vi "label_type_definition.vi"(8 "error_in":errorcluster, 10 "match_scan_code":string, 11 "scan_code":string) -> (0 "error_out":errorcluster, 2 "tooling_name":string, 3 "action":T1)   [LabVIEW 2020]
uses:
  select_action_after_parse.ctl
  control_part_number.ctl
  test_button/FGV_OBJ_test_button.ctl
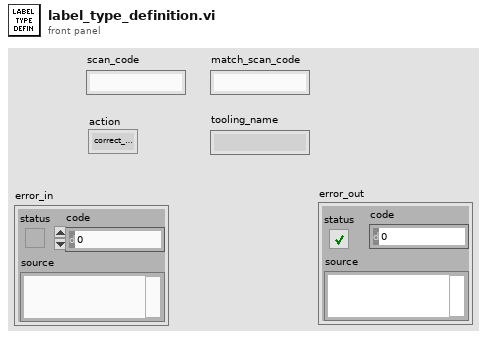
[diagram p1: front panel]
types:
  T1 = typedef "select_action_after_parse.ctl" = enum16{"correct_scan_tooling", "incorrect_scan_tooling", "correct_scan_part", "tooling_and_part_mismatch", "not_scan_tooling"}
  T2 = typedef "control_part_number.ctl" = enum16{"set_parts_number", "get_part_by_name", "set_actual_tool", "get_actual_tool"}
  T3 = typedef "FGV_OBJ_test_button.ctl" = enum16{"initialize", "set_new_login", "set_message", "enable", "disable", "disable_gray", "translate", "set_scan_tooling", "get_scan_tooling"}
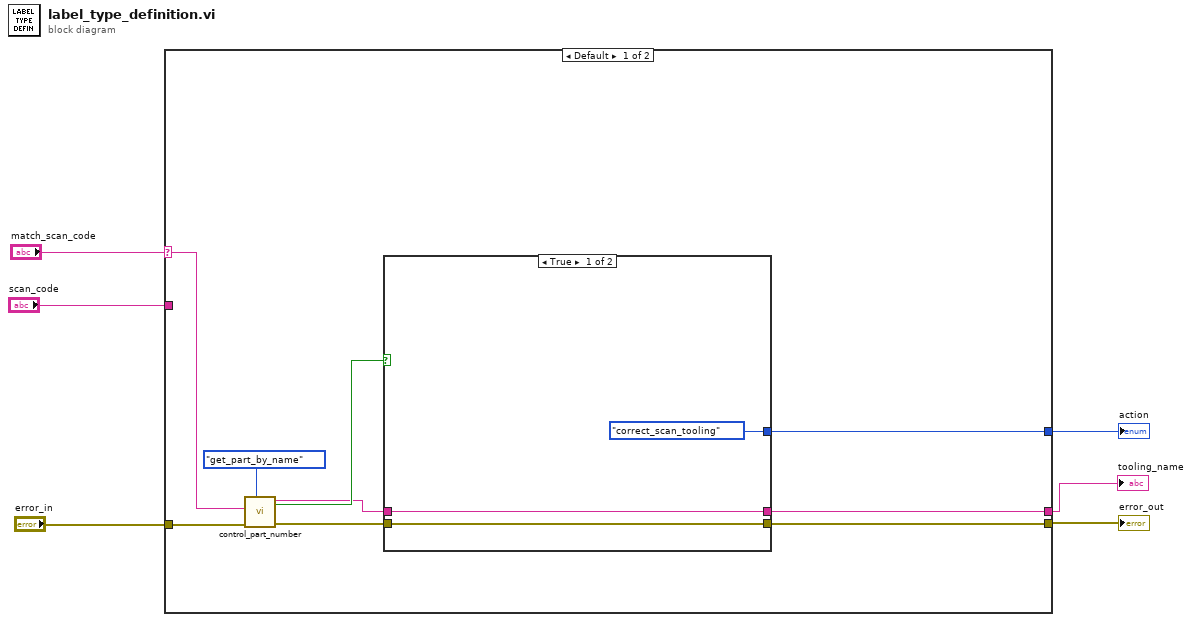
[diagram p0: block diagram]
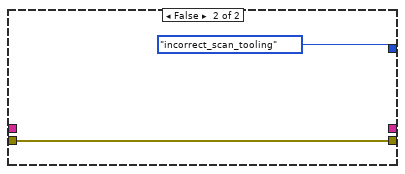
[diagram p2: hidden frame]
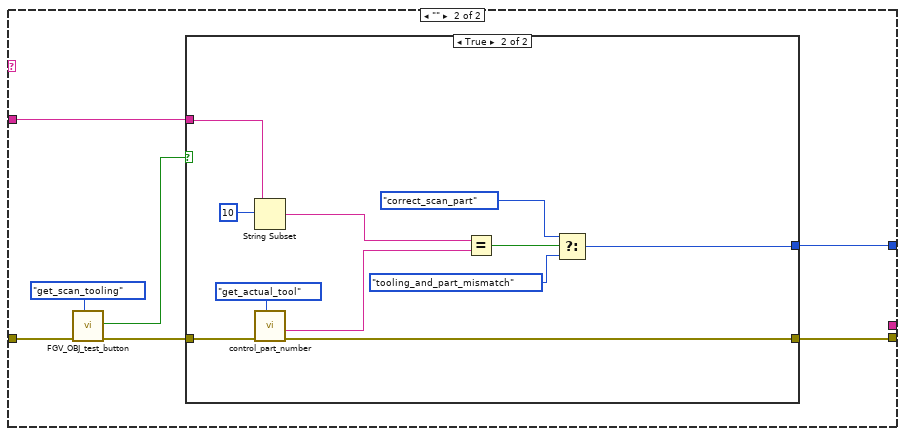
[diagram p3: hidden frame]
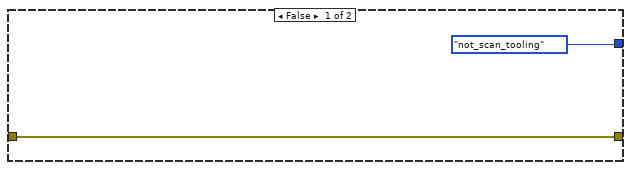
[diagram p4: hidden frame]
diagram:
  n1 = case shown="Default" "match_scan_code" {
    selector: "match_scan_code" -> [w9 _]
    tunnel: "error_in" -> [w13 w26]
    tunnel: [w15 w22] -> w4
    tunnel: "scan_code" -> [_ w24]
    tunnel: [w14 w21] -> w2
    tunnel: [w8 _] -> w1
    frame Default {
      n2 = call "control_part_number.vi"("select_for_part_number"=control_part_number."get_part_by_name", "error_in"=w13, "find_part"=w9) -> ("error_out"=w10:errorcluster, "find?"=w12:bool, "finded_part_number"=w7:string)  [unwired: 5 in, 1 out]
      n3 = case shown="True" w12 {
        tunnel: w10 -> [w18 w20]
        tunnel: [w18 w20] -> w15
        tunnel: [select_action_after_parse."correct_scan_tooling" ("action") select_action_after_parse."incorrect_scan_tooling" ("action")] -> w14
        tunnel: w7 -> [w16 _]
        tunnel: [w16 _] -> w8
        frame True {
        }
        frame False {
        }
      }
    }
    frame "" {
      n4 = call "FGV_OBJ_test_button.vi"("options"=FGV_OBJ_test_button."get_scan_tooling", "error_in"=w26) -> ("error_out"=w23:errorcluster, "scan_tooling?"=w25:bool)  [unwired: 8 in]
      n5 = case shown="True" w25 {
        tunnel: w24 -> [_ w40]
        tunnel: w23 -> [w29 w33]
        tunnel: [w29 w32] -> w22
        tunnel: [select_action_after_parse."not_scan_tooling" ("action") w37] -> w21
        frame False {
        }
        frame True {
          n6 = String Subset(string=w40, length (rest)=10) -> (substring=w36:string)  [unwired: 1 in]
          n7 = call "control_part_number.vi"("select_for_part_number"=control_part_number."get_actual_tool", "error_in"=w33) -> ("error_out"=w32:errorcluster, "actual_number_tool_output"=w35:string)  [unwired: 6 in, 2 out]
          n8 = Equal?(x=w36, y=w35) -> (x = y?=w34:bool)
          n9 = Select(t=select_action_after_parse."correct_scan_part" ("action"), s=w34, f=select_action_after_parse."tooling_and_part_mismatch" ("action")) -> (s? t:f=w37:T1)
        }
      }
    }
  }
  "error_out" <- w4
  "action" <- w2
  "tooling_name" <- w1
